vi "Dequeue Message.vi"(8 "error in (no error)":errorcluster, 11 "Zero Timeout Message Handler in":refnum<class "Zero Timeout Message Handler.lvclass">) -> (0 "error out":errorcluster, 1 "timed out?":bool, 2 "Message":refnum<class "~Message.lvclass">, 3 "Zero Timeout Message Handler out":refnum<class "Zero Timeout Message Handler.lvclass">)   [LabVIEW 2024, in "Zero Timeout Message Handler.lvlib" / "Zero Timeout Message Handler.lvclass"]
uses:
  Zero Timeout Message Handler.lvclass
  ~Message/~Message.lvclass
  Zero Timeout Message Handler.lvclass/Zero Timeout Message Handler.ctl
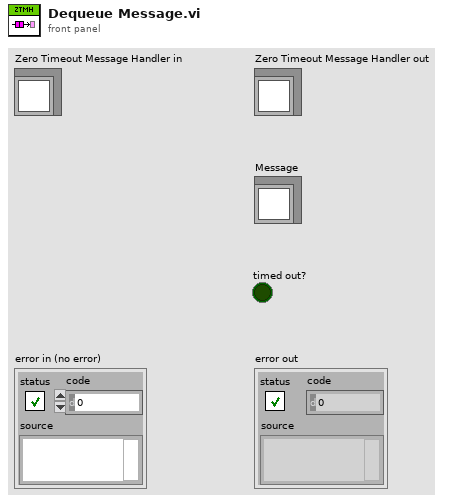
[diagram p1: front panel]
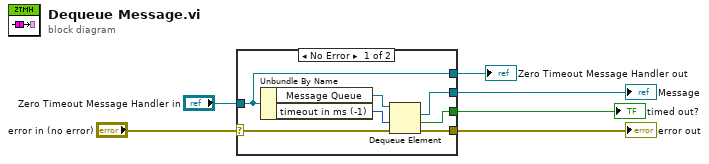
[diagram p0: block diagram]
diagram:
  n1 = case shown="No Error" "error in (no error)" {
    selector: "error in (no error)" -> [w11 w15]
    tunnel: [w10 w15] -> w5
    tunnel: [w13 w14] -> w3
    tunnel: "Zero Timeout Message Handler in" -> [w13 w14]
    tunnel: [w9 _] -> w2
    tunnel: [w7 _] -> w1
    frame No Error {
      n2 = Unbundle By Name(w13) -> ("Message Queue"=w12:refnum<queue>, "timeout in ms (-1)"=w8:i32)
      n3 = Dequeue Element(queue=w12, timeout in ms (-1)=w8, error in (no error)=w11) -> (element=w9:refnum<class "~Message.lvclass">, timed out?=w7:bool, error out=w10:errorcluster)  [unwired: 1 out]
    }
    frame Error {
    }
  }
  "error out" <- w5
  "Zero Timeout Message Handler out" <- w3
  "Message" <- w2
  "timed out?" <- w1
